vi "UserInterfaceEventHandler.vi"() -> ()   [LabVIEW 2023]
panel:
  in  "종료":bool
  in  "저장":bool caption="Blank Button"
  in  "분석":bool caption="Blank Button"
  in  "측정":bool caption="Blank Button"
  out "Count":i32
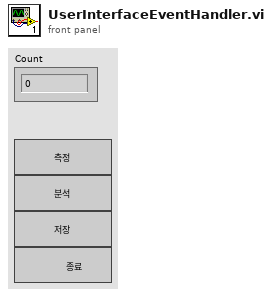
[diagram p1: front panel]
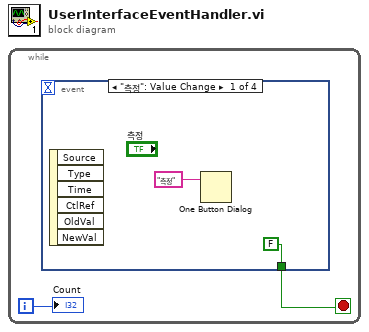
[diagram p0: block diagram]
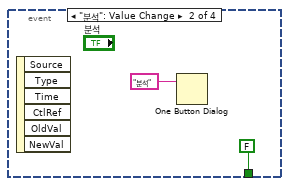
[diagram p2: hidden frame]
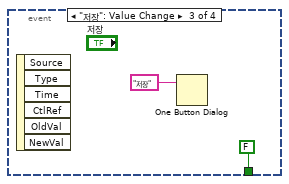
[diagram p3: hidden frame]
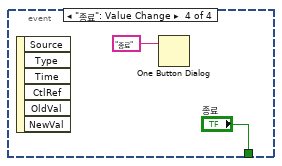
[diagram p4: hidden frame]
diagram:
  n1 = while {
    i -> [w2]
    stop <- w1 stop-if-true
    n2 = event shown="[0] \"측정\": Value Change" {
      selector: _ -> [_ _ _ _]
      dyn-events: _ -> [_ _ _ _]
      timeout: _ -> [_ _ _ _]
      tunnel: [FALSE FALSE FALSE "종료"] -> w1
      event "측정": Value Change {
        n3 = event-data() -> ()  [unwired: 1 in, 6 out]
        n4 = One Button Dialog(message="측정") -> ()  [unwired: 1 in, 1 out]
      }
      event "분석": Value Change {
        n5 = event-data() -> ()  [unwired: 1 in, 6 out]
        n6 = One Button Dialog(message="분석") -> ()  [unwired: 1 in, 1 out]
      }
      event "저장": Value Change {
        n7 = event-data() -> ()  [unwired: 1 in, 6 out]
        n8 = One Button Dialog(message="저장") -> ()  [unwired: 1 in, 1 out]
      }
      event "종료": Value Change {
        n9 = event-data() -> ()  [unwired: 1 in, 6 out]
        n10 = One Button Dialog(message="종료") -> ()  [unwired: 1 in, 1 out]
      }
    }
    "Count" <- w2
  }
